vi "grabData.vi"(8 "error in (no error)":errorcluster, 11 "URL":string) -> (0 "error out":errorcluster, 3 "body":string)   [LabVIEW 2020]
uses:
  <vilib>/httpClient/LabVIEWHTTPClient.lvlib
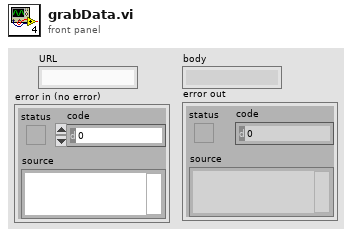
[diagram p1: front panel]
types:
  T1 = typedef "LabVIEWHTTPClient.lvlib/ClientHandle.ctl" = refnum<k1>
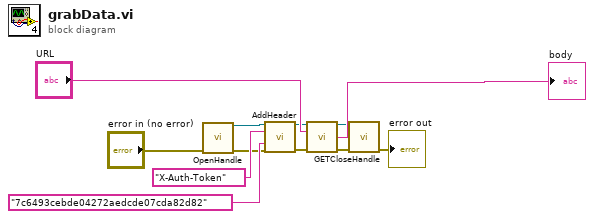
[diagram p0: block diagram]
diagram:
  n1 = call <vilib>:"OpenHandle.vi"("error in (no error)"="error in (no error)") -> ("client handle out"=w5:T1, "error out"=w3:errorcluster)  [unwired: 13 in]
  n2 = call <vilib>:"AddHeader.vi"("client handle"=w5, "header"="X-Auth-Token", "value"="7c6493cebde04272aedcde07cda82d82", "error in (no error)"=w3) -> ("client handle out"=w8:T1, "error out"=w9:errorcluster)  [unwired: 10 in]
  n3 = call <vilib>:"GET.vi"("client handle"=w8, "url"="URL", "error in (no error)"=w9) -> ("client handle out"=w4:T1, "body"=→"body":string, "error out"=w10:errorcluster)  [unwired: 9 in, 1 out]
  n4 = call <vilib>:"CloseHandle.vi"("client handle"=w4, "error in (no error)"=w10) -> ("error out"=→"error out":errorcluster)  [unwired: 13 in]
